vi "Self Configure.vi"(8 "error in":errorcluster, 11 "DAQ970 in":refnum<class "DAQ970.lvclass">) -> (0 "error out":errorcluster, 3 "DAQ970 out":refnum<class "DAQ970.lvclass">)   [LabVIEW 2019, in "DAQ970.lvlib" / "DAQ970.lvclass"]
doc: "Children of Instruments must override this routine and call the parent method. \nThis routine is implemented to allow each instrument to read its specific configuration keys and implement any default configuration settings.\n\nThis routine already calls Connect and Self Test Routines."
uses:
  Library/DAQ970.lvclass
  C:/Users/Public/Documents/Development/builds/Instruments/Instruments.lvlibp/Library/Instruments.lvclass
  Custom Controls/Configuration Keys.ctl
  builds/Instruments/Instruments.lvlibp/Accessors/Write Padding_enable.vi
  builds/Instruments/Instruments.lvlibp/Library/Instruments.lvclass
panel:
  in  "Configuration Keys":T1
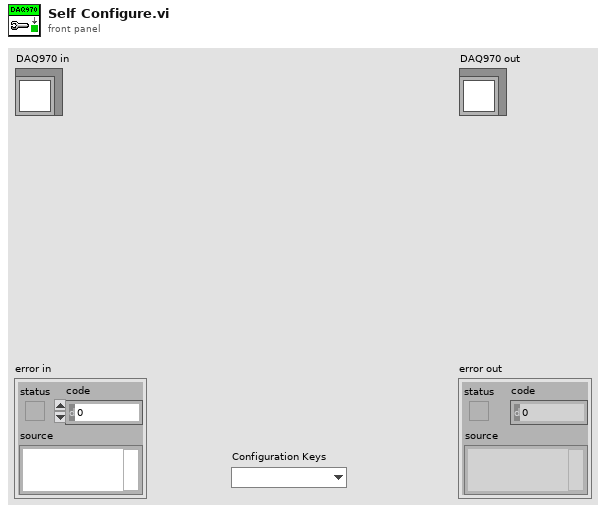
[diagram p1: front panel]
types:
  T1 = typedef "DAQ970.lvlib/DAQ970.lvclass/Configuration Keys.ctl" = enum16{""}
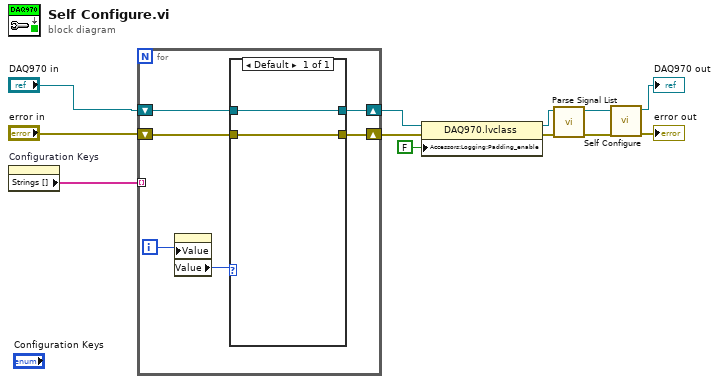
[diagram p0: block diagram]
diagram:
  n1 = property on="Configuration Keys" class="Enum (strict)"() -> ("Strings []"=w8:string[])  [unwired: 2 in, 2 out]
  n2 = for {
    shift-right: [w14] -> w5
    shift-left: "DAQ970 in" -> [w16]
    shift-right: [w13] -> w4
    shift-left: "error in" -> [w15]
    tunnel: w8 -> [_] mode=indexing
    i -> [w18]
    n3 = property on="Configuration Keys" class="Enum (strict)"("Value"=w18) -> ("Value"=w17:T1)  [unwired: 2 in, 2 out]
    n4 = case shown="Default" w17 {
      tunnel: w16 -> [w20]
      tunnel: w15 -> [w19]
      tunnel: [w20] -> w14
      tunnel: [w19] -> w13
      frame Default {
      }
    }
  }
  n5 = property class="DAQ970.lvclass"(reference=w5, error in=w4, "Accessors:Logging:Padding_enable"=FALSE ("Instrument:Logging:Padding:Enable")) -> (reference out=w3:refnum<class "DAQ970.lvclass">, error out=w2:errorcluster)
  n6 = call "Parse Signal List.vi"("error in"=w2, "DAQ970 in"=w3) -> ("error out"=w6:errorcluster, "DAQ970 out"=w7:refnum<class "DAQ970.lvclass">)  [unwired: 8 in]
  n7 = call-parent "Self Configure.vi"("error in"=w6, "Instruments in"=w7) -> ("error out"=→"error out":errorcluster, "Instruments out"=→"DAQ970 out":refnum<class "DAQ970.lvclass">)  [unwired: 8 in]
